vi "集合点.vi"() -> ()   [LabVIEW 2011]
panel:
  out "集合点2":dbl(graph)
  out "集合点1":dbl(graph)
  in  "停止":bool
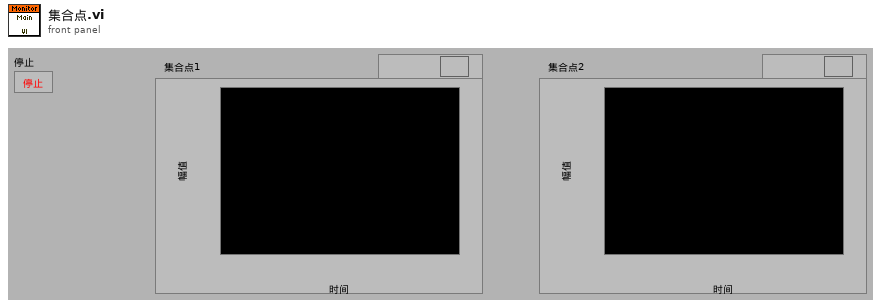
[diagram p1: front panel]
types:
  T1 = typedef "Rendezvous RefNum" = refnum<k1>
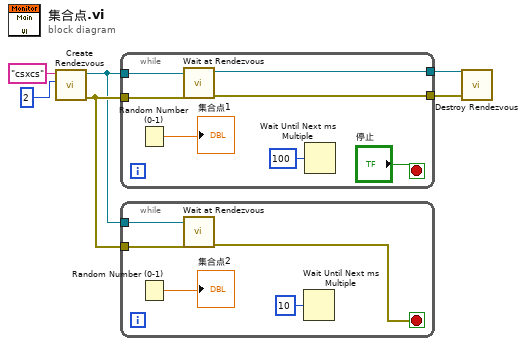
[diagram p0: block diagram]
diagram:
  n1 = call <vilib>:"Create Rendezvous.vi"("size (2)"=2, "name (unnamed)"="csxcs") -> ("error out"=w4:errorcluster, "rendezvous"=w2:T1)  [unwired: 1 in, 3 out]
  n2 = while {
    tunnel: w4 -> [w12]
    tunnel: w2 -> [w13]
    tunnel: [w11] -> w1
    tunnel: [w10] -> w3
    stop <- "停止" stop-if-true
    n3 = Random Number (0-1)() -> (number: 0 to 1=→"集合点1":dbl)
    n4 = call <vilib>:"Wait at Rendezvous.vi"("error in (no error)"=w12, "rendezvous"=w13) -> ("error out"=w11:errorcluster, "rendezvous out"=w10:T1)  [unwired: 1 in, 3 out]
    n5 = Wait Until Next ms Multiple(millisecond multiple=u32 100 ("毫秒倍数")) -> ()  [unwired: 1 out]
  }
  n6 = while {
    tunnel: w4 -> [w18]
    tunnel: w2 -> [w17]
    stop <- w16 stop-if-true
    n7 = Random Number (0-1)() -> (number: 0 to 1=→"集合点2":dbl)
    n8 = call <vilib>:"Wait at Rendezvous.vi"("error in (no error)"=w18, "rendezvous"=w17) -> ("error out"=w16:errorcluster)  [unwired: 1 in, 4 out]
    n9 = Wait Until Next ms Multiple(millisecond multiple=u32 10 ("毫秒倍数")) -> ()  [unwired: 1 out]
  }
  n10 = call <vilib>:"Destroy Rendezvous.vi"("error in (no error)"=w1, "rendezvous"=w3) -> ()  [unwired: 6 out]
